vi "Nested Aliases.vi"(11 "Actor in":refnum<class "Actor.lvclass">) -> (0 "error out":errorcluster, 2 "Nested Aliases":string[](array[string]))   [LabVIEW 2021, in "jettl.lvlib" / "Actor.lvclass"]
uses:
  Actor.lvclass
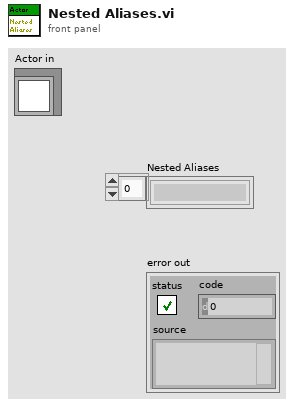
[diagram p1: front panel]
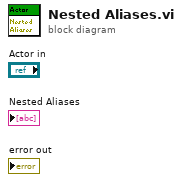
[diagram p0: block diagram]
diagram:
